vi "main.vi"() -> ()   [LabVIEW 2021]
uses:
  <vilib>/xnet/xnet.llb/XNET Frame CAN.ctl
  <vilib>/xnet/xnet.llb/XNET Frame Type CAN.ctl
  General Purpose/references.ctl
  General Purpose/measurements.ctl
  <vilib>/Platform/TimedLoop/XDataNode/timing_clust.ctl
  <vilib>/Platform/TimedLoop/XDataNode/nitl_modes.ctl
  <vilib>/Platform/TimedLoop/XDataNode/wakeup.ctl
  <instrlib>/niSync/niSync.llb/niSync Initialize (Default).vi
  <vilib>/xnet/xnet.llb/XNET Write (Frame CAN).vi
  <vilib>/xnet/xnet.llb/XNET Read (Frame CAN).vi
  <vilib>/Platform/TimedLoop/XDataNode/XDataNode.xnode
  <vilib>/Platform/TimedLoop/XDataNode/XDNodeRunTimeDep.lvlib
panel:
  out "Grandmaster Clock ID":string
  out "Synchronized":bool
  out "current time":timestamp
  in  "measurements":T1
  in  "references":T2
  out "CAN OUT":T3 {"payload" format="%x"; "timestamp" format="%<%.7X\n%x>T"; "type" items=["CAN Data"=0, "CAN Remote"=1, "CAN Bus Error"=2, "CAN 2.0 Data"=8, "CAN FD Data"=16, "CAN FD+BRS Data"=24, "J1939 Data"=192, "Delay"=224, "Log Trigger"=225, "Start Trigger"=226]; "identifier" format="%x"}
  in  "To ACT CH 4":bool
  in  "To ACT CH 3":bool
  in  "To ACT CH 2":bool
  out "Error 4":bool
  out "Fault 4":bool
  out "Error 3":bool
  out "Fault 3":bool
  out "Error 2":bool
  out "Fault 2":bool
  out "State code 4":i32
  out "State code 3":i32
  out "State code 2":i32
  out "State code 1":i32
  out "Error 1":bool
  out "Fault 1":bool
  in  "To ACT CH 1":bool
  in  "main stop":bool
  in  "Vdc4":dbl=750.0
  in  "Qac4":dbl
  in  "Vdc3":dbl=750.0
  in  "Qac3":dbl
  in  "Vdc2":dbl=750.0
  in  "Qac2":dbl
  in  "Emergency 4":bool
  in  "To IN OP  4":bool
  in  "SEND sp 4":bool
  in  "Clear 4":bool
  in  "Shutdwn 4":bool
  in  "Emergency 3":bool
  in  "To IN OP  3":bool
  in  "SEND sp 3":bool
  in  "Clear 3":bool
  in  "Shutdwn 3":bool
  in  "Emergency 2":bool
  in  "To IN OP  2":bool
  in  "SEND sp 2":bool
  in  "Clear 2":bool
  in  "Shutdwn 2":bool
  out "V slider 22":dbl(slide) caption="V-i" max=-10.0 scale=650.0..780.0 scale format="%#_4g"
  out "V slider 21":dbl(slide) caption="V-i" max=-10.0 scale=650.0..780.0 scale format="%#_4g"
  out "V slider 20":dbl(slide) caption="V-i" max=-10.0 scale=650.0..780.0 scale format="%#_4g"
  out "kW":dbl caption="Numeric" format="%#.3g"
  out "?VkVAr":dbl caption="Numeric" format="%.3g"
  out "kW":dbl caption="Numeric" format="%#.3g"
  out "?VkVAr":dbl caption="Numeric" format="%.3g"
  out "kW":dbl caption="Numeric" format="%#.3g"
  out "?VkVAr":dbl caption="Numeric" format="%.3g"
  out "OFF 4":bool
  out "ON 4":bool
  out "Ready 4":bool
  out "OFF 3":bool
  out "ON 3":bool
  out "Ready 3":bool
  out "OFF 2":bool
  out "ON 2":bool
  out "Ready 2":bool
  out "error out":errorcluster
  out "?VkVAr":dbl caption="Numeric" format="%.3g"
  out "kW":dbl caption="Numeric" format="%#.3g"
  out "V slider 19":dbl(slide) caption="V-i" max=-10.0 scale=650.0..780.0 scale format="%#_4g"
  in  "Vdc1":dbl=750.0
  out "OFF 1":bool
  out "ON 1":bool
  out "Ready 1":bool
  out "CAN IN":T3 {"payload" format="%x"; "timestamp" format="%<%.7X\n%x>T"; "type" items=["CAN Data"=0, "CAN Remote"=1, "CAN Bus Error"=2, "CAN 2.0 Data"=8, "CAN FD Data"=16, "CAN FD+BRS Data"=24, "J1939 Data"=192, "Delay"=224, "Log Trigger"=225, "Start Trigger"=226]; "identifier" format="%x"}
  in  "newfile":bool
  in  "Log period [ms]":i64=1000
  in  "Emergency 1":bool
  in  "Qac1":dbl
  in  "conv":T5
  in  "CAN [ms]":i64=1
  out "CAN with Conv":bool
  out "Measurements":bool
  in  "Shutdwn 1":bool
  in  "Clear 1":bool
  in  "SEND sp 1":bool
  in  "To IN OP 1":bool
  out "logging":bool
  # "Resource agents: AFE 1-4"
  # "package identifiers:\n1xx VSC1 \n2xx VSC2\n3xx VSC3\n4xx VSC4\n\nx0x send from agent to resource\nx02 Power setpoints\nx06 Measurements\nx9 status\n          = [state; error; alarm; OFF; Ready; ON]\n\n \n\nx1x send from resource to agent\nx10 Power measurements\nx11 Measurements\nx12 status\n          = [state; error; alarm; full; precharge; neg; 0; 0]"
  # "B18"
  # "B 22\nB19"
  # "VSC 4"
  # "B17"
  # "B21"
  # "VSC 3"
  # "B16"
  # "B20"
  # "VSC 2"
  # "B15"
  # "B19"
  # "VSC 1"
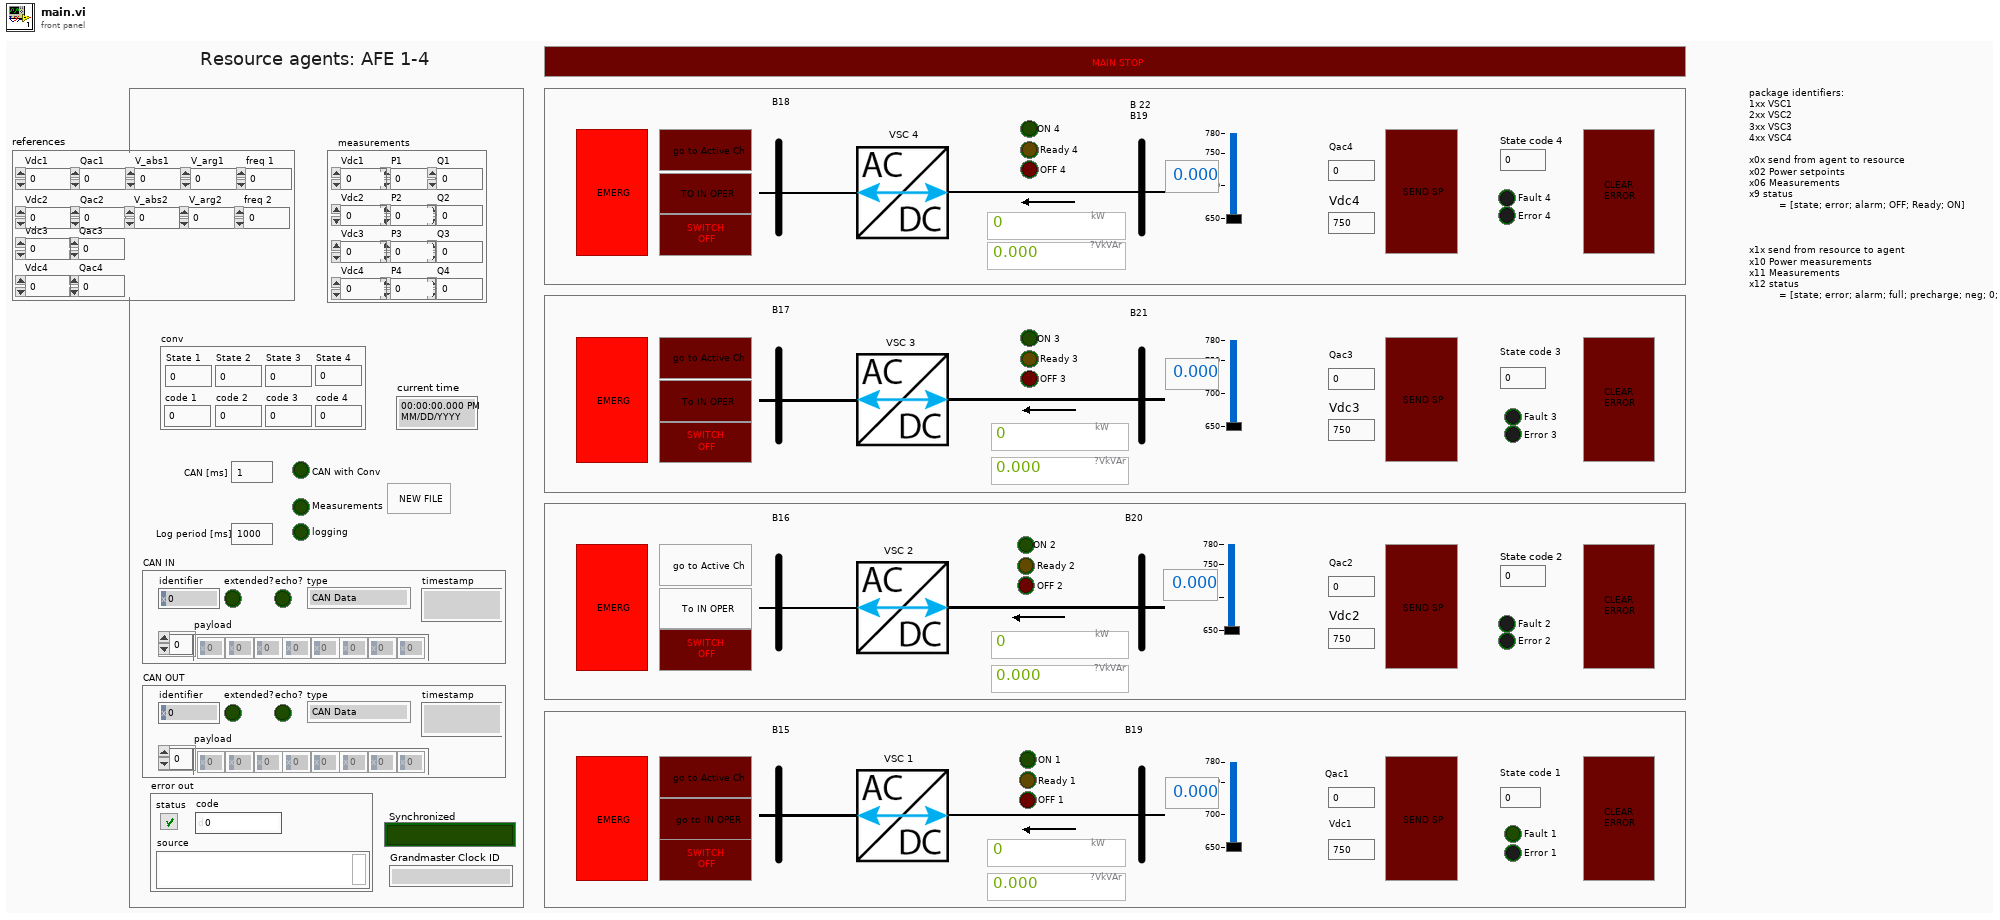
[diagram p1: front panel]
types:
  T1 = typedef "measurements.ctl" = cluster{"Vdc1":dbl, "P1":dbl, "Vdc2":dbl, "P2":dbl, "Q2":dbl, "Vdc3":dbl, "P3":dbl, "Q3":dbl, "Vdc4":dbl, "P4":dbl, "Q4":dbl, "Q1":dbl}
  T2 = typedef "references.ctl" = cluster{"Vdc1":dbl, "Vdc2":dbl, "Qac2":dbl, "Vdc3":dbl, "Qac3":dbl, "Vdc4":dbl, "Qac4":dbl, "Qac1":dbl, "V_arg2":dbl, "V_abs2":dbl, "V_abs1":dbl, "V_arg1":dbl, "freq 1":dbl, "freq 2":dbl}
  T3 = typedef "XNET Frame CAN.ctl" = cluster{"timestamp":timestamp, "payload":u8[], "identifier":u32, "type":T4, "extended?":bool, "echo?":bool}
  T4 = typedef "XNET Frame Type CAN.ctl" = u8
  T5 = cluster{"State 1":dbl, "code 1":dbl, "code 2":dbl, "code 3":dbl, "code 4":dbl, "State 2":dbl, "State 3":dbl, "State 4":dbl}
  T6 = cluster{"Frame In":refnum<k21>, "Frame Out":refnum<k21>}
  T7 = typedef "XDNodeRunTimeDep.lvlib/timing_clust.ctl" = cluster{"Expected End [f-1]":u64, "Actual End [f-1]":u64, "Finished Late? [f-1]":bool, "Expected End [i-1]":u64, "Actual End [i-1]":u64, "Finished Late? [i-1]":bool, "Expected Start [i]":u64, "Actual Start [i]":u64, "Expected Start [f]":u64, "Actual Start [f]":u64, "Source Name":string, "Structure Name":string, "Period":i64, "Deadline":i64, "Offset":i64, "Start":i64, "Priority":i32, "Timeout":i32, "Mode":T8, "Wakeup Reason":T9, "Error":errorcluster, "Source Type":string, "Secondary Source Type":string, "Global End Time":u64, "Global Start Time":u64, "Frame Duration":u64, "Iteration Duration":u64, "Assigned CPU":i32, "I/O Scan Engine Mode":u32}
  T8 = typedef "XDNodeRunTimeDep.lvlib/nitl_modes.ctl" = enum32{"No Change", "Process missed periods, maintain original phase", "Discard missed periods, maintain original phase", "Process missed periods, ignore original phase", "Discard missed periods, ignore original phase"}
  T9 = typedef "XDNodeRunTimeDep.lvlib/wakeup.ctl" = enum32{"Normal", "Aborted", "Asynchronous wakeup", "Timing source error", "Timed loop error", "Timeout"}
  T10 = cluster{"date string":string, "time string":string, "Vdc1":dbl, "P1":dbl, "Q1":dbl, "Vdc2":dbl, "P2":dbl, "Q2":dbl, "Vdc3":dbl, "P3":dbl, "Q3":dbl, "Vdc4":dbl, "P4":dbl, "Q4":dbl}
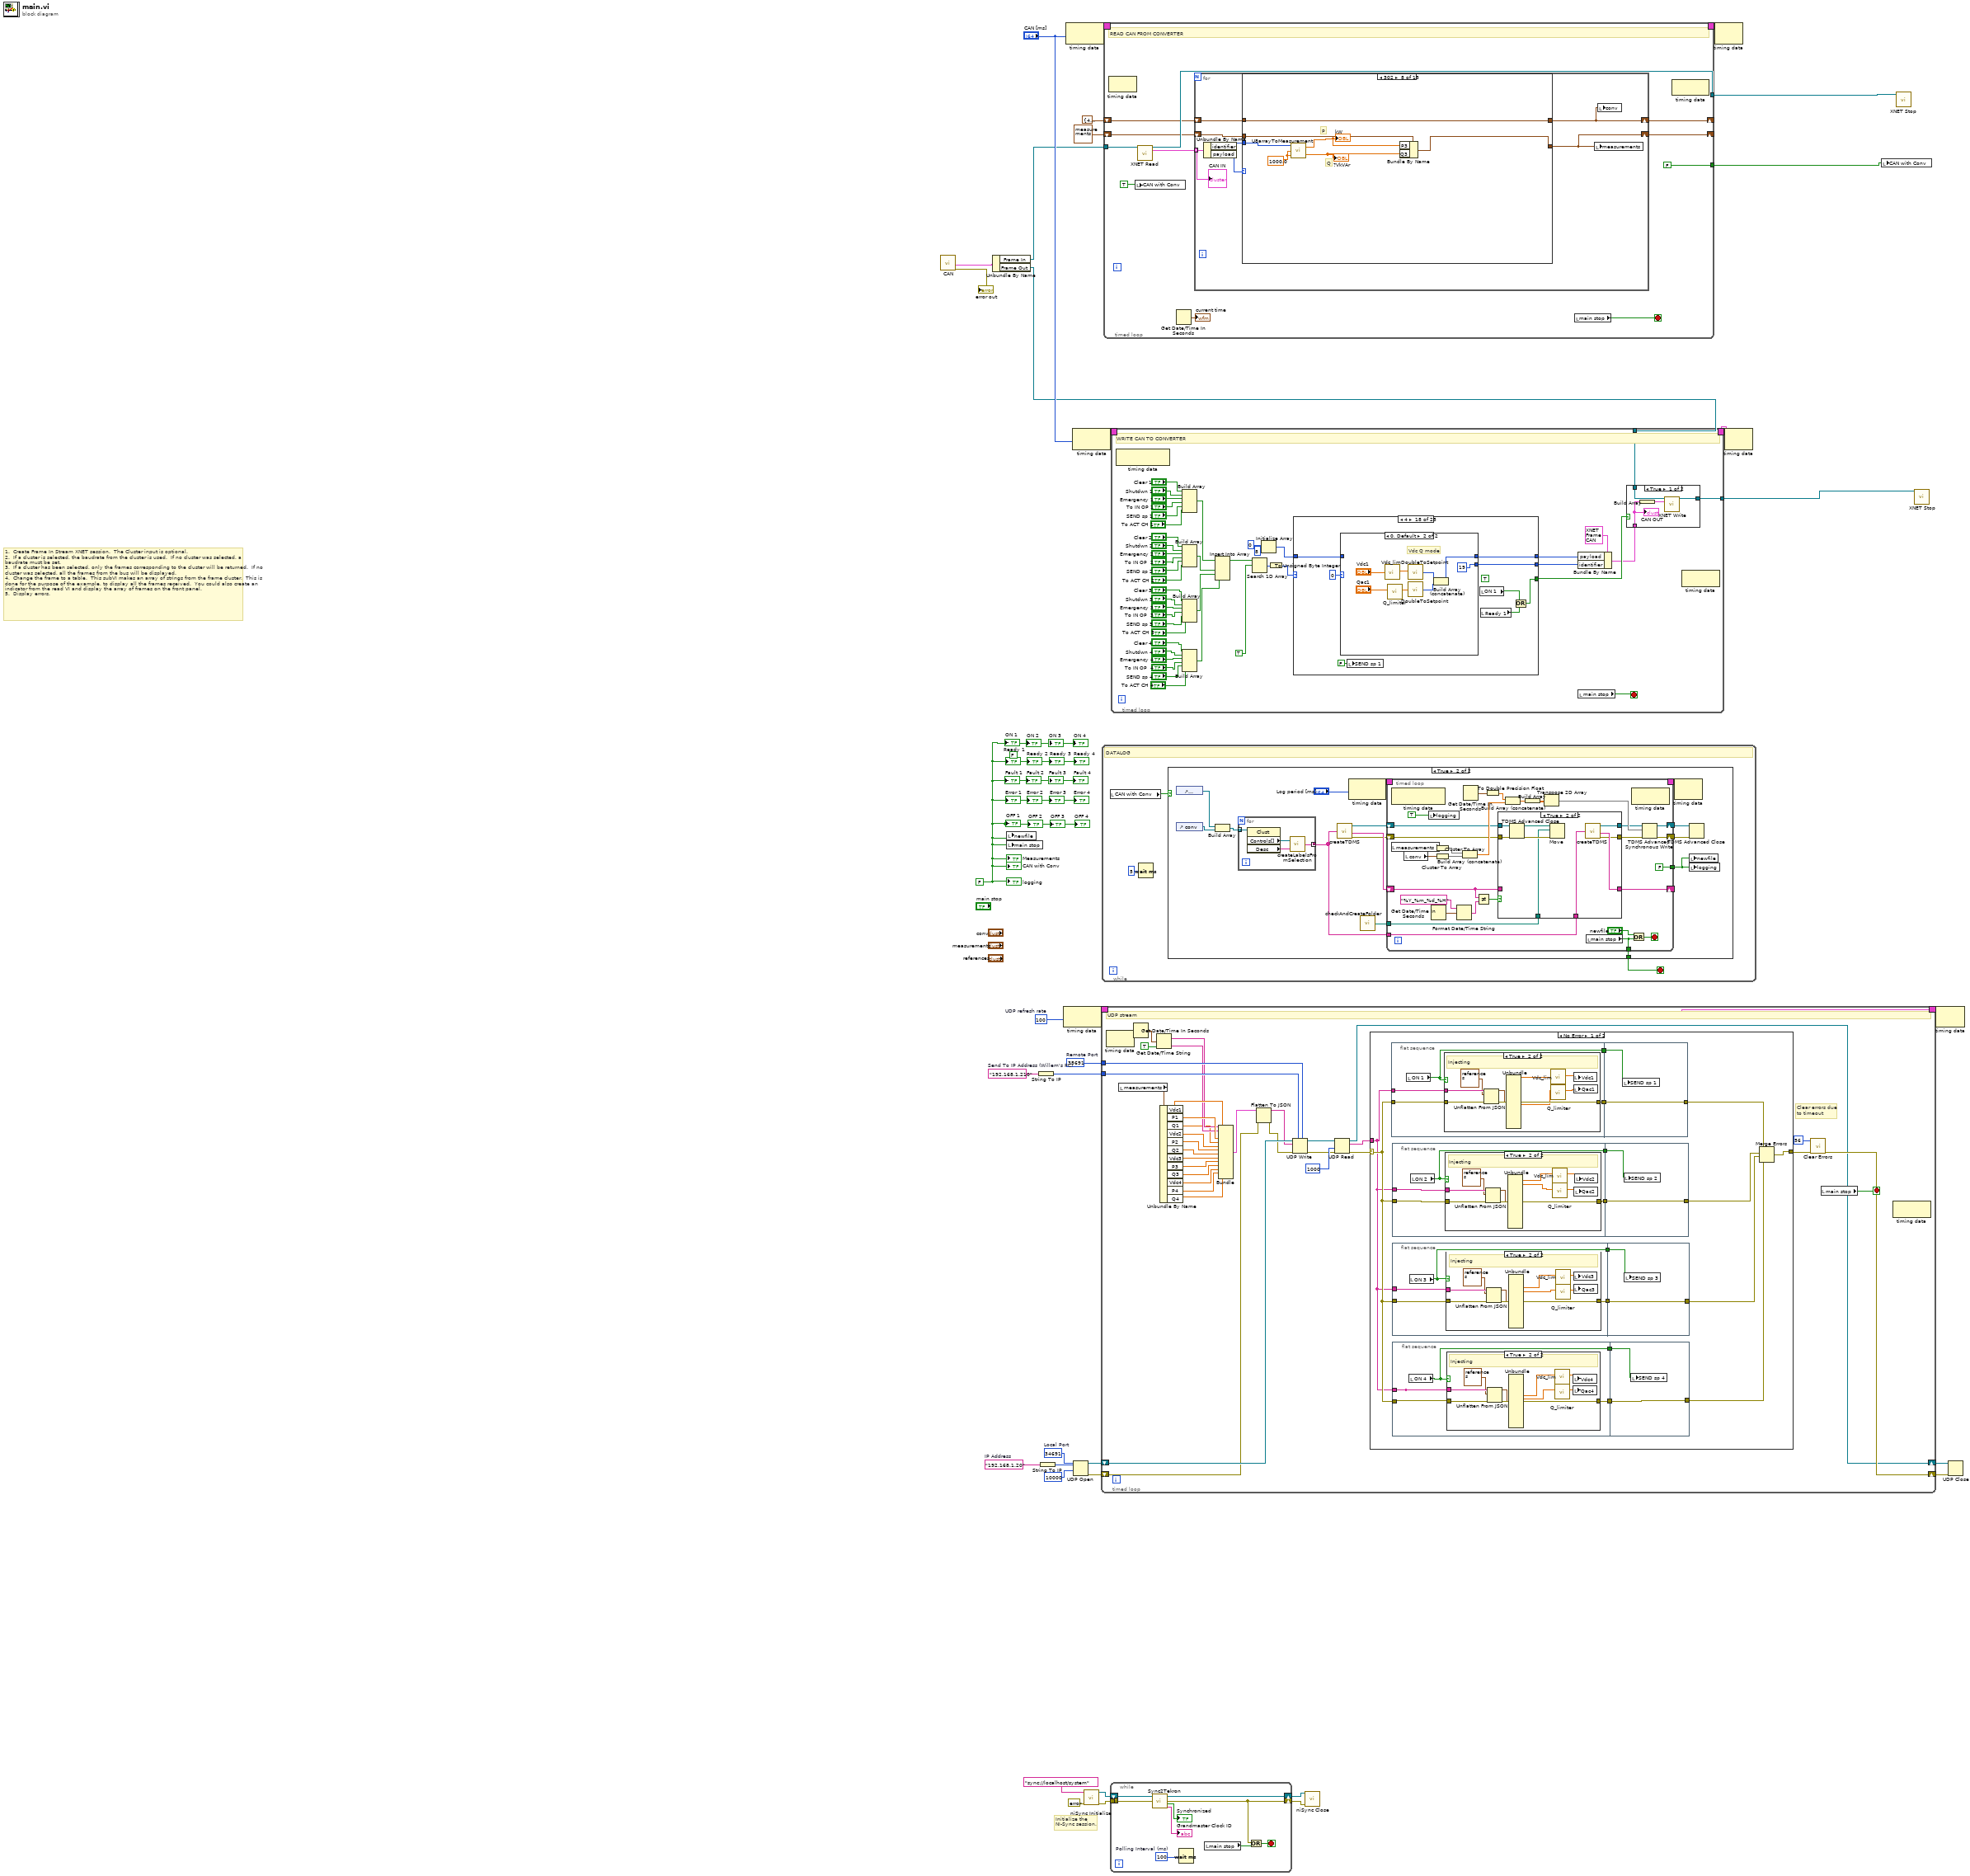
[diagram p0: block diagram]
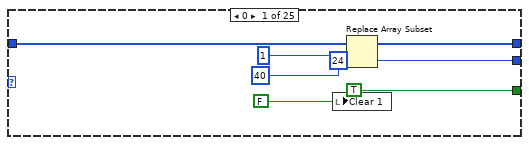
[diagram p8: hidden frame]
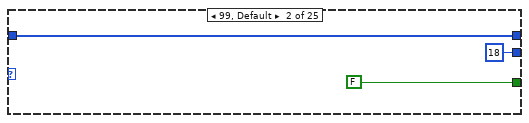
[diagram p9: hidden frame]
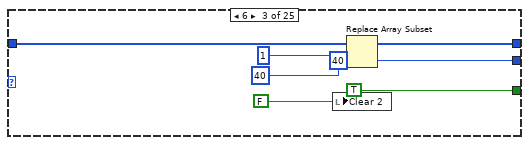
[diagram p10: hidden frame]
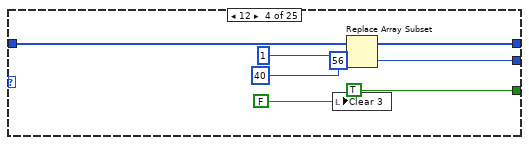
[diagram p11: hidden frame]
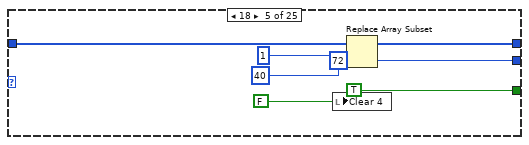
[diagram p12: hidden frame]
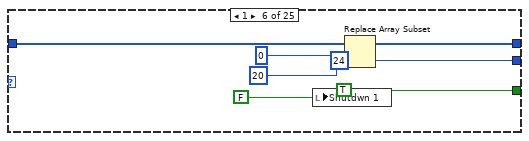
[diagram p13: hidden frame]
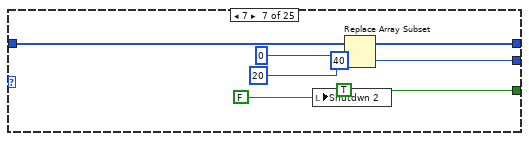
[diagram p14: hidden frame]
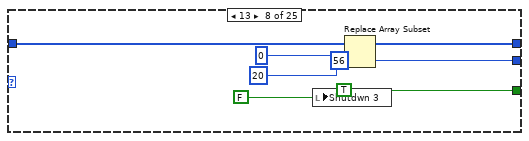
[diagram p15: hidden frame]
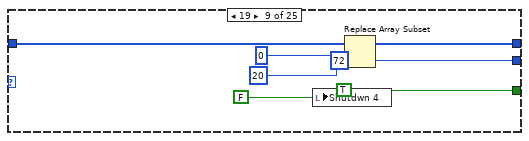
[diagram p16: hidden frame]
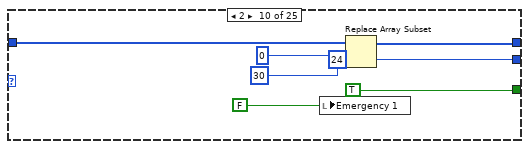
[diagram p17: hidden frame]
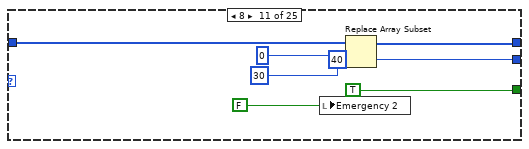
[diagram p18: hidden frame]
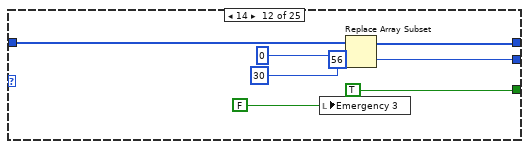
[diagram p19: hidden frame]
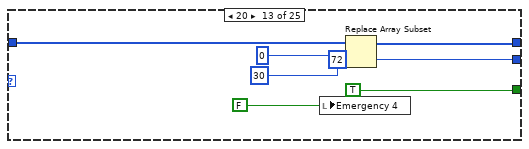
[diagram p20: hidden frame]
diagram:
  (unwired) FALSE ("ON 2")
  (unwired) FALSE ("ON 2")
  w14 = i64 100  # UDP refresh rate
  w19 = u16 34691  # Local Port
  w20 = "192.168.1.20"  # IP Address
  w10 = u16 35691  # Remote Port
  w18 = "192.168.1.210"  # Send To IP Address (Willem's PC)
  w7 = FALSE
  # "Initialize the\nNI-Sync session."
  # "1.  Create Frame In Stream XNET session.  The Cluster input is optional.  \n2.  If a cluster is selected, the baudrate from the cluster is used.  If no cluster was selected, a baudrate must be set.\n3.  If a cluster has been selected, only the frames corresponding to the cluster will be returned.  If no cluster was selected, all the frames from the bus will be displayed.\n4.  Change the frame to a table.  This subVI makes an array of strings from the frame cluster.  This is done for the purpose of the example, to display all the frames received.  You could also create an indicator from the read VI and display the array of frames on the front panel. \n5.  Display errors."
  n1 = call "CAN.vi"() -> ("error out"=→"error out":errorcluster, "CAN"=w9:T6)  [unwired: 10 in]
  n2 = Unbundle By Name(w9) -> ("Frame In"=w28:refnum<k21>, "Frame Out"=w31:refnum<k21>)
  n3 = local write "newfile"(w7) -> ()
  n4 = local write "main stop"(w7) -> ()
  n5 = String To IP(1:w18) -> (0:w11:u32)
  n6 = String To IP(1:w20) -> (0:w21:u32)
  n7 = node-c288(w14) -> (w23:T7)
  n8 = node-c288("CAN [ms]") -> (w30:T7)
  n9 = node-c288("CAN [ms]") -> (w25:T7)
  n10 = UDP Open(7:w21, 9:10000 ("timeout ms (25000)"), 11:w19) -> (port=w13:refnum<k16>, 0:w12:errorcluster)  [unwired: 2 in, 1 out]
  n11 = call-poly <instrlib>:"niSync Initialize.vi"("error in (no error)"=errorcluster {"status"=FALSE, "code"=0, "source"=""}, "resource name"=tag "sync://localhost/system" ("NI-Sync Resource")) -> ("error out"=w4:errorcluster, "instrument handle out"=w1:refnum<k15>)  [unwired: 8 in]
  n12 = timed-loop {
    timing: w23 -> [_]
    timing-out: [_] -> w22
    shift-right: [w53] -> w17
    shift-left: w13 -> [w69]
    shift-right: [w59] -> w16
    shift-left: w12 -> [w66]
    tunnel: w11 -> [w63]
    tunnel: w10 -> [w62]
    stop <- w61 stop-if-true
    # "Clear errors due\nto timeout"
    # "UDP stream"
    n13 = node-c288() -> ()  [unwired: 1 in, 1 out]
    n14 = local read "measurements"() -> (w48:T1)
    n15 = Get Date/Time In Seconds() -> (seconds since 1Jan1904=w52:timestamp)
    n16 = Get Date/Time String(seconds (now)=w52, want seconds? (F)=TRUE) -> (date string=w51:string, time string=w50:string)  [unwired: 1 in]
    n17 = Unbundle By Name(w48) -> ("Vdc1"=w68:dbl, "P1"=w67:dbl, "Q1"=w47:dbl, "Vdc2"=w46:dbl, "P2"=w44:dbl, "Q2"=w43:dbl, "Vdc3"=w42:dbl, "P3"=w41:dbl, "Q3"=w40:dbl, "Vdc4"=w39:dbl, "P4"=w38:dbl, "Q4"=w37:dbl)
    n18 = Bundle("date string"=w51, "time string"=w50, "Vdc1"=w68, "P1"=w67, "Q1"=w47, "Vdc2"=w46, "P2"=w44, "Q2"=w43, "Vdc3"=w42, "P3"=w41, "Q3"=w40, "Vdc4"=w39, "P4"=w38, "Q4"=w37) -> (w45:T10)  [unwired: 1 in]
    n19 = Flatten To JSON(anything=w45, error in (no error)=w66) -> (JSON string=w64:string, 11:w65:errorcluster)  [unwired: 1 in]
    n20 = UDP Write(address=w63, port or service name=w62, connection ID=w69, data in=w64, 8:w65) -> (error out=w55:errorcluster, 3:w54:refnum<k16>)  [unwired: 1 in]
    n21 = UDP Read(connection ID=w54, timeout ms (25000)=1000, 8:w55) -> (data out=w58:string, error out=w57:errorcluster, 3:w53:refnum<k16>)  [unwired: 1 in, 2 out]
    n22 = case shown="No Error" w57 {
      selector: w57 -> [w82 w149]
      tunnel: w58 -> [w81 _]
      tunnel: [w83 w149] -> w36
      frame No Error {
        n23 = flat-sequence {
          tunnel: w81 -> [w136]
          tunnel: w82 -> [w135]
          tunnel: [w134] -> w84
          tunnel: [w133] -> w70
          tunnel: w84 -> [w148]
          tunnel: [w148] -> w80
          tunnel: w70 -> [w147]
          frame #0 {
            n24 = local read "ON 1"() -> (w133:bool)
            n25 = case shown="True" w133 {
              tunnel: w136 -> [_ w146]
              tunnel: w135 -> [w137 w145]
              tunnel: [w137 w144] -> w134
              frame False {
                # "Injecting"
              }
              frame True {
                # "Injecting"
                n26 = Unflatten From JSON(JSON string=w146, type and defaults=T2 {"Vdc1"=0.0, "Vdc2"=0.0, "Qac2"=0.0, "Vdc3"=0.0, "Qac3"=0.0, "Vdc4"=0.0, "Qac4"=0.0, "Qac1"=0.0, "V_arg2"=0.0, "V_abs2"=0.0, "V_abs1"=0.0, "V_arg1"=0.0, "freq 1"=0.0, "freq 2"=0.0} ("ref"), error in (no error)=w145) -> (value=w143:T2, error out=w144:errorcluster)  [unwired: 4 in]
                n27 = Unbundle(w143) -> ("Vdc1"=w140:dbl, "Qac1"=w138:dbl)  [unwired: 12 out]
                n28 = call "Vdc_lim.vi"("IN Vdc"=w140) -> ("OUT Vdc"=w141:dbl)  [unwired: 10 in]
                n29 = call "Q_limiter.vi"("IN Q"=w138) -> ("OUT Q"=w139:dbl)  [unwired: 10 in]
                n30 = local write "Vdc1"(w141) -> ()
                n31 = local write "Qac1"(w139) -> ()
              }
            }
          }
          frame #1 {
            n32 = local write "SEND sp 1"(w147) -> ()
          }
        }
        n33 = flat-sequence {
          tunnel: w82 -> [w120]
          tunnel: w81 -> [w118]
          tunnel: [w119] -> w74
          tunnel: [w117] -> w71
          tunnel: [w132] -> w77
          tunnel: w74 -> [w132]
          tunnel: w71 -> [w131]
          frame #0 {
            n34 = local read "ON 2"() -> (w117:bool)
            n35 = case shown="True" w117 {
              tunnel: w118 -> [_ w130]
              tunnel: w120 -> [w121 w129]
              tunnel: [w121 w128] -> w119
              frame False {
                # "Injecting"
              }
              frame True {
                # "Injecting"
                n36 = Unflatten From JSON(JSON string=w130, type and defaults=T2 {"Vdc1"=0.0, "Vdc2"=0.0, "Qac2"=0.0, "Vdc3"=0.0, "Qac3"=0.0, "Vdc4"=0.0, "Qac4"=0.0, "Qac1"=0.0, "V_arg2"=0.0, "V_abs2"=0.0, "V_abs1"=0.0, "V_arg1"=0.0, "freq 1"=0.0, "freq 2"=0.0} ("ref"), error in (no error)=w129) -> (value=w127:T2, error out=w128:errorcluster)  [unwired: 4 in]
                n37 = Unbundle(w127) -> ("Vdc2"=w124:dbl, "Qac2"=w122:dbl)  [unwired: 12 out]
                n38 = call "Vdc_lim.vi"("IN Vdc"=w124) -> ("OUT Vdc"=w125:dbl)  [unwired: 10 in]
                n39 = call "Q_limiter.vi"("IN Q"=w122) -> ("OUT Q"=w123:dbl)  [unwired: 10 in]
                n40 = local write "Qac2"(w123) -> ()
                n41 = local write "Vdc2"(w125) -> ()
              }
            }
          }
          frame #1 {
            n42 = local write "SEND sp 2"(w131) -> ()
          }
        }
        n43 = flat-sequence {
          tunnel: w82 -> [w104]
          tunnel: w81 -> [w102]
          tunnel: [w103] -> w75
          tunnel: [w101] -> w72
          tunnel: [w116] -> w78
          tunnel: w75 -> [w116]
          tunnel: w72 -> [w115]
          frame #0 {
            n44 = local read "ON 3"() -> (w101:bool)
            n45 = case shown="True" w101 {
              tunnel: w102 -> [_ w114]
              tunnel: w104 -> [w105 w113]
              tunnel: [w105 w112] -> w103
              frame False {
                # "Injecting"
              }
              frame True {
                # "Injecting"
                n46 = Unflatten From JSON(JSON string=w114, type and defaults=T2 {"Vdc1"=0.0, "Vdc2"=0.0, "Qac2"=0.0, "Vdc3"=0.0, "Qac3"=0.0, "Vdc4"=0.0, "Qac4"=0.0, "Qac1"=0.0, "V_arg2"=0.0, "V_abs2"=0.0, "V_abs1"=0.0, "V_arg1"=0.0, "freq 1"=0.0, "freq 2"=0.0} ("ref"), error in (no error)=w113) -> (value=w111:T2, error out=w112:errorcluster)  [unwired: 4 in]
                n47 = Unbundle(w111) -> ("Vdc3"=w108:dbl, "Qac3"=w106:dbl)  [unwired: 12 out]
                n48 = call "Vdc_lim.vi"("IN Vdc"=w108) -> ("OUT Vdc"=w109:dbl)  [unwired: 10 in]
                n49 = call "Q_limiter.vi"("IN Q"=w106) -> ("OUT Q"=w107:dbl)  [unwired: 10 in]
                n50 = local write "Vdc3"(w109) -> ()
                n51 = local write "Qac3"(w107) -> ()
              }
            }
          }
          frame #1 {
            n52 = local write "SEND sp 3"(w115) -> ()
          }
        }
        n53 = flat-sequence {
          tunnel: w82 -> [w88]
          tunnel: [w86] -> _
          tunnel: w81 -> [w86]
          tunnel: [w87] -> w76
          tunnel: [w85] -> w73
          tunnel: [w100] -> w79
          tunnel: w76 -> [w100]
          tunnel: w73 -> [w99]
          frame #0 {
            n54 = local read "ON 4"() -> (w85:bool)
            n55 = case shown="True" w85 {
              tunnel: w86 -> [_ w98]
              tunnel: w88 -> [w89 w97]
              tunnel: [w89 w96] -> w87
              frame False {
                # "Injecting"
              }
              frame True {
                # "Injecting"
                n56 = Unflatten From JSON(JSON string=w98, type and defaults=T2 {"Vdc1"=0.0, "Vdc2"=0.0, "Qac2"=0.0, "Vdc3"=0.0, "Qac3"=0.0, "Vdc4"=0.0, "Qac4"=0.0, "Qac1"=0.0, "V_arg2"=0.0, "V_abs2"=0.0, "V_abs1"=0.0, "V_arg1"=0.0, "freq 1"=0.0, "freq 2"=0.0} ("ref"), error in (no error)=w97) -> (value=w95:T2, error out=w96:errorcluster)  [unwired: 4 in]
                n57 = Unbundle(w95) -> ("Vdc4"=w92:dbl, "Qac4"=w91:dbl)  [unwired: 12 out]
                n58 = call "Vdc_lim.vi"("IN Vdc"=w92) -> ("OUT Vdc"=w93:dbl)  [unwired: 10 in]
                n59 = call "Q_limiter.vi"("IN Q"=w91) -> ("OUT Q"=w90:dbl)  [unwired: 10 in]
                n60 = local write "Vdc4"(w93) -> ()
                n61 = local write "Qac4"(w90) -> ()
              }
            }
          }
          frame #1 {
            n62 = local write "SEND sp 4"(w99) -> ()
          }
        }
        n63 = Merge Errors(w80, w77, w78, w79) -> (w83:errorcluster)
      }
      frame Error {
      }
    }
    n64 = call <vilib>:"Clear Errors.vi"("error in (no error)"=w36, "specific error code to clear (0: all)"=56) -> ("error out"=w59:errorcluster)  [unwired: 4 in, 1 out]
    n65 = local read "main stop"() -> (w61:bool)
    n66 = node-c288() -> ()  [unwired: 1 in, 1 out]
  }
  n67 = while {
    stop <- w154 stop-if-true
    # "DATALOG"
    n68 = local read "CAN with Conv"() -> (w152:bool)
    n69 = Wait (ms)(milliseconds to wait=u32 5) -> ()  [unwired: 1 out]
    n70 = case shown="True" w152 {
      selector: w152 -> [w155 _]
      tunnel: [w155 w168] -> w154
      frame False {
      }
      frame True {
        n71 = control-ref of="measurements"() -> (w156:refnum<vi>)
        n72 = control-ref of="conv"() -> (w161:refnum<vi>)
        n73 = Build Array(w156, w161) -> (w160:refnum<vi>[])
        n74 = for {
          tunnel: [w172] -> w159 mode=concatenating
          tunnel: w160 -> [w171] mode=indexing
          n75 = property class="Clust"(reference=w171) -> ("Controls[]"=w174:refnum<vi>[], "Desc"=w173:string)  [unwired: 1 in, 2 out]
          n76 = call "createLabelsFromSelection.vi"("log_from"=w173, "Controls[]"=w174) -> ("labels_to_log"=w172:string[])
        }
        n77 = call "createTDMS.vi"("channel name(s)"=w159) -> ("Ref"=w157:refnum<k34>, "hour"=w163:string, "error out"=w158:errorcluster)  [unwired: 3 in]
        n78 = node-c288("Log period [ms]") -> (w170:T7)
        n79 = call "checkAndCreateFolder.vi"() -> ("dup path"=w162:path)  [unwired: 1 in]
        n80 = timed-loop {
          timing: w170 -> [_]
          timing-out: [_] -> w169
          tunnel: [w194] -> w168
          tunnel: [FALSE ("logging")] -> w164
          shift-right: [w185] -> _
          shift-left: w163 -> [w184]
          tunnel: w162 -> [w183]
          tunnel: w159 -> [w182]
          shift-right: [w195] -> w165
          shift-left: w158 -> [w176]
          shift-right: [w203] -> w166
          shift-left: w157 -> [w175]
          stop <- w197 stop-if-true
          n81 = node-c288() -> ()  [unwired: 1 in, 1 out]
          n82 = local read "measurements"() -> (w181:T1)
          n83 = local read "conv"() -> (w180:T5)
          n84 = local write "logging"(TRUE ("logging")) -> ()
          n85 = Get Date/Time In Seconds() -> (seconds since 1Jan1904=w188:timestamp)
          n86 = Cluster To Array(cluster=w181) -> (array=w179:dbl[])
          n87 = Cluster To Array(cluster=w180) -> (array=w178:dbl[])
          n88 = Format Date/Time String(time format string (%c)="%Y_%m_%d_%H", seconds (now)=w188) -> (date/time string=w186:string)  [unwired: 1 in]
          n89 = Build Array (concatenate)(w179, w178) -> (w177:dbl[])
          n90 = Get Date/Time In Seconds() -> (seconds since 1Jan1904=w199:timestamp)
          n91 = Not Equal?(x=w184, y=w186) -> (x != y?=w187:bool)
          n92 = To Double Precision Float(number=w199) -> (double precision float=w198:dbl)
          n93 = case shown="True" w187 {
            tunnel: w175 -> [w206 w215]
            tunnel: [w206 w209] -> w191
            tunnel: w176 -> [w205 w214]
            tunnel: [w205 w207] -> w190
            tunnel: [w204 w208] -> w185
            tunnel: w184 -> [w204 _]
            tunnel: w183 -> [_ w211]
            tunnel: w182 -> [_ w210]
            frame False {
            }
            frame True {
              n94 = TDMS Advanced Close(8:w214, 11:w215) -> (0:w213:errorcluster, 3:w212:path)  [unwired: 2 in]
              n95 = Move(source path=w212, error in=w213, 10:w211) -> ()  [unwired: 2 in, 3 out]
              n96 = call "createTDMS.vi"("channel name(s)"=w210) -> ("Ref"=w209:refnum<k34>, "hour"=w208:string, "error out"=w207:errorcluster)  [unwired: 3 in]
            }
          }
          n97 = Build Array (concatenate)(w198, w177) -> (w202:dbl[])
          n98 = Build Array(w202) -> (w201:dbl[][])
          n99 = Transpose 2D Array(2D array=w201) -> (transposed array=w200:dbl[][])
          n100 = local read "main stop"() -> (w194:bool)
          n101 = node-c288() -> ()  [unwired: 1 in, 1 out]
          n102 = Or(x="newfile", y=w194) -> (x .or. y?=w197:bool)
          n103 = TDMS Advanced Synchronous Write(8:w190, 10:w200, 11:w191) -> (0:w195:errorcluster, 3:w203:refnum<k34>)
        }
        n104 = node-c288(w169) -> ()  [unwired: 1 out]
        n105 = TDMS Advanced Close(8:w165, 11:w166) -> ()  [unwired: 2 in, 2 out]
        n106 = local write "newfile"(w164) -> ()
        n107 = local write "logging"(w164) -> ()
      }
    }
  }
  n108 = timed-loop {
    timing: w30 -> [_]
    timing-out: [_] -> w29
    tunnel: w28 -> [w225]
    tunnel: [w231] -> w35
    shift-right: [w226] -> _
    shift-left: T5 {"State 1"=4.0, "code 1"=0.0, "code 2"=0.0, "code 3"=0.0, "code 4"=0.0, "State 2"=4.0, "State 3"=4.0, "State 4"=4.0} ("Conv 2") -> [w230]
    tunnel: [FALSE ("stop CAN")] -> w32
    shift-right: [w223] -> _
    shift-left: T1 {"Vdc1"=0.0, "P1"=0.0, "Vdc2"=0.0, "P2"=0.0, "Q2"=0.0, "Vdc3"=0.0, "P3"=0.0, "Q3"=0.0, "Vdc4"=0.0, "P4"=0.0, "Q4"=0.0, "Q1"=0.0} ("measurements 2") -> [w224]
    stop <- w229 stop-if-true
    # "READ CAN FROM CONVERTER"
    n109 = node-c288() -> ()  [unwired: 1 in, 1 out]
    n110 = local write "CAN with Conv"(TRUE) -> ()
    n111 = call-poly <vilib>:"XNET Read.vi"("session in"=w225) -> ("session out"=w231:refnum<k21>, "data"=w232:T3[])  [unwired: 11 in, 2 out]
    n112 = Get Date/Time In Seconds() -> (seconds since 1Jan1904=→"current time":timestamp)
    n113 = for {
      tunnel: w232 -> [w237] mode=indexing
      shift-right: [w235] -> w226
      shift-left: w230 -> [w236]
      shift-right: [w233] -> w223
      shift-left: w224 -> [w234]
      n114 = Unbundle By Name(w237) -> ("identifier"=w239:u32, "payload"=w238:u8[])
      n115 = case shown="302" w239 {
        tunnel: w238 -> [_ w246 w271 w296 w321 w348 w355 w362 w369 w374 w382 w390 w398]
        tunnel: w236 -> [w241 w254 w279 w304 w329 w346 w353 w360 w367 w372 w378 w387 w395]
        tunnel: [w241 w253 w278 w303 w328 w346 w353 w360 w367 w372 w378 w387 w395] -> w235
        tunnel: w234 -> [w240 w243 w268 w293 w319 w344 w349 w356 w363 w370 w377 w386 w393]
        tunnel: [w240 w244 w269 w294 w320 w345 w350 w357 w364 w371 w376 w385 w394] -> w233
        frame 0, Default {
        }
        frame 25 {
          w242 = 1.0 ("factor 1")
          n116 = Index Array(array=w246, index=0) -> (element=w247:u8)
          n117 = call "U8arrayToMeasurement.vi"("factor 2"=w242, "factor 1"=w242, "payload"=w246) -> ("Meas 2"=w245:dbl)  [unwired: 1 out]
          "V slider 19" <- w245
          n118 = Index Array(array=w246, index=1) -> (element=w250:u8)
          n119 = Index Array(array=w246, index=2) -> (element=w249:u8)
          n120 = Join Numbers(hi=w250, lo=w249) -> ((hi.lo)=w248:u16)
          "State code 1" <- w248
          n121 = Bundle By Name(cluster=w243, "Vdc1"=w245) -> (w244:T1)
          n122 = case shown="5" w247 {
            frame 5 {
              w257 = FALSE ("Fault 1")
              n123 = local write "Fault 1"(TRUE ("Fault 1")) -> ()
              n124 = local write "Error 1"(w257) -> ()
              n125 = local write "OFF 1"(w257) -> ()
              n126 = local write "Ready 1"(w257) -> ()
              n127 = local write "ON 1"(w257) -> ()
            }
            frame 1 {
              w258 = FALSE ("Fault 1")
              n128 = local write "Fault 1"(w258) -> ()
              n129 = local write "Error 1"(TRUE ("Error 1")) -> ()
              n130 = local write "OFF 1"(w258) -> ()
              n131 = local write "Ready 1"(w258) -> ()
              n132 = local write "ON 1"(w258) -> ()
            }
            frame 2 {
              w261 = FALSE ("Fault 1")
              n133 = local write "Fault 1"(w261) -> ()
              n134 = local write "Error 1"(w261) -> ()
              n135 = local write "OFF 1"(TRUE ("OFF 1")) -> ()
              n136 = local write "Ready 1"(w261) -> ()
              n137 = local write "ON 1"(w261) -> ()
            }
            frame 3 {
              w263 = FALSE ("Fault 1")
              n138 = local write "Fault 1"(w263) -> ()
              n139 = local write "Error 1"(w263) -> ()
              n140 = local write "OFF 1"(w263) -> ()
              n141 = local write "Ready 1"(TRUE ("Ready 1")) -> ()
              n142 = local write "ON 1"(w263) -> ()
            }
            frame 4 {
              w265 = FALSE ("Fault 1")
              n143 = local write "Fault 1"(w265) -> ()
              n144 = local write "Error 1"(w265) -> ()
              n145 = local write "OFF 1"(w265) -> ()
              n146 = local write "Ready 1"(w265) -> ()
              n147 = local write "ON 1"(TRUE ("ON 1")) -> ()
            }
            frame 99, Default {
              w266 = FALSE ("Fault 1")
              n148 = local write "Fault 1"(w266) -> ()
              n149 = local write "Error 1"(w266) -> ()
              n150 = local write "OFF 1"(w266) -> ()
              n151 = local write "Ready 1"(w266) -> ()
              n152 = local write "ON 1"(w266) -> ()
            }
          }
          n153 = Bundle By Name(cluster=w254, "State 1"=w247, "code 1"=w248) -> (w253:T5)
        }
        frame 41 {
          w267 = 1.0 ("factor 1")
          n154 = call "U8arrayToMeasurement.vi"("factor 2"=w267, "factor 1"=w267, "payload"=w271) -> ("Meas 2"=w270:dbl)  [unwired: 1 out]
          "V slider 20" <- w270
          n155 = Index Array(array=w271, index=0) -> (element=w277:u8)
          n156 = Index Array(array=w271, index=1) -> (element=w274:u8)
          n157 = Index Array(array=w271, index=2) -> (element=w273:u8)
          n158 = Join Numbers(hi=w274, lo=w273) -> ((hi.lo)=w272:u16)
          "State code 2" <- w272
          n159 = Bundle By Name(cluster=w268, "Vdc2"=w270) -> (w269:T1)
          n160 = case shown="5" w277 {
            frame 5 {
              w282 = FALSE ("Fault 1")
              n161 = local write "Fault 2"(TRUE ("Fault 1")) -> ()
              n162 = local write "Error 2"(w282) -> ()
              n163 = local write "OFF 2"(w282) -> ()
              n164 = local write "Ready 2"(w282) -> ()
              n165 = local write "ON 2"(w282) -> ()
            }
            frame 1 {
              w283 = FALSE ("Fault 1")
              n166 = local write "Fault 2"(w283) -> ()
              n167 = local write "Error 2"(TRUE ("Error 1")) -> ()
              n168 = local write "OFF 2"(w283) -> ()
              n169 = local write "Ready 2"(w283) -> ()
              n170 = local write "ON 2"(w283) -> ()
            }
            frame 2 {
              w286 = FALSE ("Fault 1")
              n171 = local write "Fault 2"(w286) -> ()
              n172 = local write "Error 2"(w286) -> ()
              n173 = local write "OFF 2"(TRUE ("OFF 1")) -> ()
              n174 = local write "Ready 2"(w286) -> ()
              n175 = local write "ON 2"(w286) -> ()
            }
            frame 3 {
              w288 = FALSE ("Fault 1")
              n176 = local write "Fault 2"(w288) -> ()
              n177 = local write "Error 2"(w288) -> ()
              n178 = local write "OFF 2"(w288) -> ()
              n179 = local write "Ready 2"(TRUE ("Ready 1")) -> ()
              n180 = local write "ON 2"(w288) -> ()
            }
            frame 4 {
              w290 = FALSE ("Fault 1")
              n181 = local write "Fault 2"(w290) -> ()
              n182 = local write "Error 2"(w290) -> ()
              n183 = local write "OFF 2"(w290) -> ()
              n184 = local write "Ready 2"(w290) -> ()
              n185 = local write "ON 2"(TRUE ("ON 1")) -> ()
            }
            frame 99, Default {
              w291 = FALSE ("Fault 1")
              n186 = local write "Fault 2"(w291) -> ()
              n187 = local write "Error 2"(w291) -> ()
              n188 = local write "OFF 2"(w291) -> ()
              n189 = local write "Ready 2"(w291) -> ()
              n190 = local write "ON 2"(w291) -> ()
            }
          }
          n191 = Bundle By Name(cluster=w279, "State 2"=w277, "code 2"=w272) -> (w278:T5)
        }
        frame 57 {
          w292 = 1.0 ("factor 1")
          n192 = Index Array(array=w296, index=0) -> (element=w302:u8)
          n193 = Index Array(array=w296, index=1) -> (element=w299:u8)
          n194 = Index Array(array=w296, index=2) -> (element=w298:u8)
          n195 = call "U8arrayToMeasurement.vi"("factor 2"=w292, "factor 1"=w292, "payload"=w296) -> ("Meas 2"=w295:dbl)  [unwired: 1 out]
          "V slider 21" <- w295
          n196 = Join Numbers(hi=w299, lo=w298) -> ((hi.lo)=w297:u16)
          "State code 3" <- w297
          n197 = case shown="5" w302 {
            frame 5 {
              w307 = FALSE ("Fault 1")
              n198 = local write "Fault 3"(TRUE ("Fault 1")) -> ()
              n199 = local write "Error 3"(w307) -> ()
              n200 = local write "OFF 3"(w307) -> ()
              n201 = local write "Ready 3"(w307) -> ()
              n202 = local write "ON 3"(w307) -> ()
            }
            frame 1 {
              w308 = FALSE ("Fault 1")
              n203 = local write "Fault 3"(w308) -> ()
              n204 = local write "Error 3"(TRUE ("Error 1")) -> ()
              n205 = local write "OFF 3"(w308) -> ()
              n206 = local write "Ready 3"(w308) -> ()
              n207 = local write "ON 3"(w308) -> ()
            }
            frame 2 {
              w311 = FALSE ("Fault 1")
              n208 = local write "Fault 3"(w311) -> ()
              n209 = local write "Error 3"(w311) -> ()
              n210 = local write "OFF 3"(TRUE ("OFF 1")) -> ()
              n211 = local write "Ready 3"(w311) -> ()
              n212 = local write "ON 3"(w311) -> ()
            }
            frame 3 {
              w313 = FALSE ("Fault 1")
              n213 = local write "Fault 3"(w313) -> ()
              n214 = local write "Error 3"(w313) -> ()
              n215 = local write "OFF 3"(w313) -> ()
              n216 = local write "Ready 3"(TRUE ("Ready 1")) -> ()
              n217 = local write "ON 3"(w313) -> ()
            }
            frame 4 {
              w315 = FALSE ("Fault 1")
              n218 = local write "Fault 3"(w315) -> ()
              n219 = local write "Error 3"(w315) -> ()
              n220 = local write "OFF 3"(w315) -> ()
              n221 = local write "Ready 3"(w315) -> ()
              n222 = local write "ON 3"(TRUE ("ON 1")) -> ()
            }
            frame 99, Default {
              w316 = FALSE ("Fault 1")
              n223 = local write "Fault 3"(w316) -> ()
              n224 = local write "Error 3"(w316) -> ()
              n225 = local write "OFF 3"(w316) -> ()
              n226 = local write "Ready 3"(w316) -> ()
              n227 = local write "ON 3"(w316) -> ()
            }
          }
          n228 = Bundle By Name(cluster=w293, "Vdc3"=w295) -> (w294:T1)
          n229 = Bundle By Name(cluster=w304, "State 3"=w302, "code 3"=w297) -> (w303:T5)
        }
        frame 73 {
          w317 = 1.0 ("factor 1")
          n230 = Index Array(array=w321, index=0) -> (element=w327:u8)
          n231 = Index Array(array=w321, index=1) -> (element=w324:u8)
          n232 = Index Array(array=w321, index=2) -> (element=w323:u8)
          n233 = Join Numbers(hi=w324, lo=w323) -> ((hi.lo)=w322:u16)
          "State code 4" <- w322
          n234 = call "U8arrayToMeasurement.vi"("factor 2"=w317, "factor 1"=w317, "payload"=w321) -> ("Meas 2"=w318:dbl)  [unwired: 1 out]
          "V slider 22" <- w318
          n235 = case shown="5" w327 {
            frame 5 {
              w332 = FALSE ("Fault 1")
              n236 = local write "Fault 4"(TRUE ("Fault 1")) -> ()
              n237 = local write "Error 4"(w332) -> ()
              n238 = local write "OFF 4"(w332) -> ()
              n239 = local write "Ready 4"(w332) -> ()
              n240 = local write "ON 4"(w332) -> ()
            }
            frame 1 {
              w333 = FALSE ("Fault 1")
              n241 = local write "Fault 4"(w333) -> ()
              n242 = local write "Error 4"(TRUE ("Error 1")) -> ()
              n243 = local write "OFF 4"(w333) -> ()
              n244 = local write "Ready 4"(w333) -> ()
              n245 = local write "ON 4"(w333) -> ()
            }
            frame 2 {
              w336 = FALSE ("Fault 1")
              n246 = local write "Fault 4"(w336) -> ()
              n247 = local write "Error 4"(w336) -> ()
              n248 = local write "OFF 4"(TRUE ("OFF 1")) -> ()
              n249 = local write "Ready 4"(w336) -> ()
              n250 = local write "ON 4"(w336) -> ()
            }
            frame 3 {
              w338 = FALSE ("Fault 1")
              n251 = local write "Fault 4"(w338) -> ()
              n252 = local write "Error 4"(w338) -> ()
              n253 = local write "OFF 4"(w338) -> ()
              n254 = local write "Ready 4"(TRUE ("Ready 1")) -> ()
              n255 = local write "ON 4"(w338) -> ()
            }
            frame 4 {
              w340 = FALSE ("Fault 1")
              n256 = local write "Fault 4"(w340) -> ()
              n257 = local write "Error 4"(w340) -> ()
              n258 = local write "OFF 4"(w340) -> ()
              n259 = local write "Ready 4"(w340) -> ()
              n260 = local write "ON 4"(TRUE ("ON 1")) -> ()
            }
            frame 99, Default {
              w341 = FALSE ("Fault 1")
              n261 = local write "Fault 4"(w341) -> ()
              n262 = local write "Error 4"(w341) -> ()
              n263 = local write "OFF 4"(w341) -> ()
              n264 = local write "Ready 4"(w341) -> ()
              n265 = local write "ON 4"(w341) -> ()
            }
          }
          n266 = Bundle By Name(cluster=w319, "Vdc4"=w318) -> (w320:T1)
          n267 = Bundle By Name(cluster=w329, "State 4"=w327, "code 4"=w322) -> (w328:T5)
        }
        frame 258 {
          w347 = 1000.0 ("factor 1")
          # "Q"
          # "P"
          n268 = call "U8arrayToMeasurement.vi"("factor 2"=w347, "factor 1"=w347, "payload"=w348) -> ("Meas 2"=w342:dbl, "Meas 1"=w343:dbl)
          "kW" <- w343
          "?VkVAr" <- w342
          n269 = Bundle By Name(cluster=w344, "P1"=w343, "Q1"=w342) -> (w345:T1)
        }
        frame 514 {
          w354 = 1000.0 ("factor 1")
          # "Q"
          # "P"
          n270 = call "U8arrayToMeasurement.vi"("factor 2"=w354, "factor 1"=w354, "payload"=w355) -> ("Meas 2"=w351:dbl, "Meas 1"=w352:dbl)
          "kW" <- w352
          "?VkVAr" <- w351
          n271 = Bundle By Name(cluster=w349, "P2"=w352, "Q2"=w351) -> (w350:T1)
        }
        frame 770 {
          w361 = 1000.0 ("factor 1")
          # "Q"
          # "P"
          n272 = call "U8arrayToMeasurement.vi"("factor 2"=w361, "factor 1"=w361, "payload"=w362) -> ("Meas 2"=w358:dbl, "Meas 1"=w359:dbl)
          "kW" <- w359
          "?VkVAr" <- w358
          n273 = Bundle By Name(cluster=w356, "P3"=w359, "Q3"=w358) -> (w357:T1)
        }
        frame 1026 {
          w368 = 1000.0 ("factor 1")
          # "Q"
          # "P"
          n274 = call "U8arrayToMeasurement.vi"("factor 2"=w368, "factor 1"=w368, "payload"=w369) -> ("Meas 2"=w365:dbl, "Meas 1"=w366:dbl)
          "kW" <- w366
          "?VkVAr" <- w365
          n275 = Bundle By Name(cluster=w363, "P4"=w366, "Q4"=w365) -> (w364:T1)
        }
        frame 262 {
          w375 = 1.0 ("factor 1")
          n276 = call "U8arrayToMeasurement.vi"("factor 2"=w375, "factor 1"=w375, "payload"=w374) -> ("Meas 1"=w373:dbl)  [unwired: 1 out]
          n277 = Bundle By Name(cluster=w370, "Vdc1"=w373) -> (w371:T1)
        }
        frame 518 {
          w383 = 1.0 ("factor 1")
          # "Vdc"
          n278 = call "U8arrayToMeasurement.vi"("factor 2"=w383, "factor 1"=w383, "payload"=w382) -> ("Meas 2"=w380:dbl, "Meas 1"=w381:dbl)
          n279 = Add(x=w381, y=w380) -> (x+y=w379:dbl)
          n280 = Bundle By Name(cluster=w377, "Vdc2"=w379) -> (w376:T1)
        }
        frame 774 {
          w391 = 1.0 ("factor 1")
          # "Vdc"
          n281 = call "U8arrayToMeasurement.vi"("factor 2"=w391, "factor 1"=w391, "payload"=w390) -> ("Meas 2"=w388:dbl, "Meas 1"=w389:dbl)
          n282 = Add(x=w389, y=w388) -> (x+y=w384:dbl)
          n283 = Bundle By Name(cluster=w386, "Vdc3"=w384) -> (w385:T1)
        }
        frame 1030 {
          w399 = 1.0 ("factor 1")
          # "Vdc"
          n284 = call "U8arrayToMeasurement.vi"("factor 2"=w399, "factor 1"=w399, "payload"=w398) -> ("Meas 2"=w396:dbl, "Meas 1"=w397:dbl)
          n285 = Add(x=w397, y=w396) -> (x+y=w392:dbl)
          n286 = Bundle By Name(cluster=w393, "Vdc4"=w392) -> (w394:T1)
        }
      }
      n287 = local write "measurements"(w233) -> ()
      n288 = local write "conv"(w235) -> ()
      "CAN IN" <- w237
    }
    n289 = local read "main stop"() -> (w229:bool)
    n290 = node-c288() -> ()  [unwired: 1 in, 1 out]
  }
  n291 = while {
    shift-right: [w404] -> w2
    shift-left: _ -> [w406]
    shift-right: [w405] -> w3
    shift-left: w1 -> [w407]
    tunnel: w4 -> [_]
    stop <- w409 stop-if-true
    w410 = u32 100  # Polling Interval (ms)
    n292 = call "Sync2Tekron.vi"("instrument handle in"=w407, "error in (no error)"=w406) -> ("instrument handle out"=w405:refnum<k15>, "error out"=w404:errorcluster, "Synchronized"=→"Synchronized":bool, "Grandmaster Clock ID"=→"Grandmaster Clock ID":string)  [unwired: 5 in]
    n293 = Wait (ms)(milliseconds to wait=w410) -> ()  [unwired: 1 out]
    n294 = local read "main stop"() -> (w408:bool)
    n295 = Or(x=w404, y=w408) -> (x .or. y?=w409:bool)
  }
  n296 = timed-loop {
    tunnel: w31 -> [w445]
    tunnel: [w444] -> w34
    timing: w25 -> [_]
    timing-out: [_] -> w24
    stop <- w443 stop-if-true
    # "WRITE CAN TO CONVERTER"
    n297 = node-c288() -> ()  [unwired: 1 in, 1 out]
    n298 = Build Array("Clear 1", "Shutdwn 1", "Emergency 1", "To IN OP 1", "SEND sp 1", "To ACT CH 1") -> (w419:bool[])
    n299 = Build Array("Clear 2", "Shutdwn 2", "Emergency 2", "To IN OP  2", "SEND sp 2", "To ACT CH 2") -> (w418:bool[])
    n300 = Build Array("Clear 3", "Shutdwn 3", "Emergency 3", "To IN OP  3", "SEND sp 3", "To ACT CH 3") -> (w417:bool[])
    n301 = Build Array("Clear 4", "Shutdwn 4", "Emergency 4", "To IN OP  4", "SEND sp 4", "To ACT CH 4") -> (w416:bool[])
    n302 = Insert Into Array(array=w419, new element #1=w418, new element #2=w417, new element #3=w416) -> (w415:bool[])  [unwired: 1 in]
    n303 = Search 1D Array(1D array=w415, element=TRUE) -> (index of element=w437:i32)  [unwired: 1 in]
    n304 = Initialize Array(u8 0, 8 ("dimension size")) -> (w451:u8[])
    n305 = To Unsigned Byte Integer(number=w437) -> (unsigned 8bit integer=w441:u8)
    n306 = case shown="4" w441 {
      tunnel: [w465 w468 w475 w482 w489 w496 w503 w510 w517 w523 w530 w537 w544 w551 w558 w565 w572 w582 w600 w618 w636 w651 w658 w665 w672] -> w450
      tunnel: [u32 24 ("identifier") u32 18 ("identifier") u32 40 ("identifier") u32 56 ("identifier") u32 72 ("identifier") u32 24 ("identifier") u32 40 ("identifier") u32 56 ("identifier") u32 72 ("identifier") u32 24 ("identifier") u32 40 ("identifier") u32 56 ("identifier") u32 72 ("identifier") u32 24 ("identifier") u32 40 ("identifier") u32 56 ("identifier") u32 72 ("identifier") w580 w598 w616 w634 u32 24 ("identifier") u32 40 ("identifier") u32 56 ("identifier") u32 72 ("identifier")] -> w449
      tunnel: w451 -> [w463 w468 w473 w480 w487 w495 w502 w509 w516 w524 w531 w538 w545 w552 w559 w566 w573 w579 w597 w615 w633 w652 w659 w666 w673]
      tunnel: [TRUE FALSE TRUE TRUE TRUE TRUE TRUE TRUE TRUE TRUE TRUE TRUE TRUE TRUE TRUE TRUE TRUE w577 w593 w612 w629 TRUE TRUE TRUE TRUE] -> w447
      frame 0 {
        n307 = local write "Clear 1"(FALSE ("Clear")) -> ()
        n308 = Replace Array Subset(array=w463, new element=u8 40 ("new element/subarray"), index=1) -> (w465:u8[])
      }
      frame 99, Default {
      }
      frame 6 {
        n309 = local write "Clear 2"(FALSE ("Clear")) -> ()
        n310 = Replace Array Subset(array=w473, new element=u8 40 ("new element/subarray"), index=1) -> (w475:u8[])
      }
      frame 12 {
        n311 = local write "Clear 3"(FALSE ("Clear")) -> ()
        n312 = Replace Array Subset(array=w480, new element=u8 40 ("new element/subarray"), index=1) -> (w482:u8[])
      }
      frame 18 {
        n313 = local write "Clear 4"(FALSE ("Clear")) -> ()
        n314 = Replace Array Subset(array=w487, new element=u8 40 ("new element/subarray"), index=1) -> (w489:u8[])
      }
      frame 1 {
        n315 = local write "Shutdwn 1"(FALSE ("Shutdwn")) -> ()
        n316 = Replace Array Subset(array=w495, new element=u8 20 ("new element/subarray"), index=0) -> (w496:u8[])
      }
      frame 7 {
        n317 = local write "Shutdwn 2"(FALSE ("Shutdwn")) -> ()
        n318 = Replace Array Subset(array=w502, new element=u8 20 ("new element/subarray"), index=0) -> (w503:u8[])
      }
      frame 13 {
        n319 = local write "Shutdwn 3"(FALSE ("Shutdwn")) -> ()
        n320 = Replace Array Subset(array=w509, new element=u8 20 ("new element/subarray"), index=0) -> (w510:u8[])
      }
      frame 19 {
        n321 = local write "Shutdwn 4"(FALSE ("Shutdwn")) -> ()
        n322 = Replace Array Subset(array=w516, new element=u8 20 ("new element/subarray"), index=0) -> (w517:u8[])
      }
      frame 2 {
        n323 = local write "Emergency 1"(FALSE ("Idc cmd")) -> ()
        n324 = Replace Array Subset(array=w524, new element=u8 30 ("new element/subarray"), index=0) -> (w523:u8[])
      }
      frame 8 {
        n325 = local write "Emergency 2"(FALSE ("Idc cmd")) -> ()
        n326 = Replace Array Subset(array=w531, new element=u8 30 ("new element/subarray"), index=0) -> (w530:u8[])
      }
      frame 14 {
        n327 = local write "Emergency 3"(FALSE ("Idc cmd")) -> ()
        n328 = Replace Array Subset(array=w538, new element=u8 30 ("new element/subarray"), index=0) -> (w537:u8[])
      }
      frame 20 {
        n329 = local write "Emergency 4"(FALSE ("Idc cmd")) -> ()
        n330 = Replace Array Subset(array=w545, new element=u8 30 ("new element/subarray"), index=0) -> (w544:u8[])
      }
      frame 3 {
        n331 = local write "To IN OP 1"(FALSE ("Idc cmd")) -> ()
        n332 = Replace Array Subset(array=w552, new element=u8 2 ("new element/subarray"), index=0) -> (w551:u8[])
      }
      frame 9 {
        n333 = local write "To IN OP  2"(FALSE ("Idc cmd")) -> ()
        n334 = Replace Array Subset(array=w559, new element=u8 2 ("new element/subarray"), index=0) -> (w558:u8[])
      }
      frame 15 {
        n335 = local write "To IN OP  3"(FALSE ("Idc cmd")) -> ()
        n336 = Replace Array Subset(array=w566, new element=u8 2 ("new element/subarray"), index=0) -> (w565:u8[])
      }
      frame 21 {
        n337 = local write "To IN OP  4"(FALSE ("Idc cmd")) -> ()
        n338 = Replace Array Subset(array=w573, new element=u8 2 ("new element/subarray"), index=0) -> (w572:u8[])
      }
      frame 4 {
        (unwired) TRUE
        n339 = case shown="0, Default" u8 0 ("Con_State") {
          tunnel: [w583 w589] -> w582
          tunnel: [u32 16 ("identifier") u32 19 ("identifier")] -> w580
          tunnel: w579 -> [w583 _]
          frame 6 {
            # "PQ mode"
          }
          frame 0, Default {
            # "Vdc Q mode"
            n340 = call "Vdc_lim.vi"("IN Vdc"="Vdc1") -> ("OUT Vdc"=w587:dbl)  [unwired: 10 in]
            n341 = call "Q_limiter.vi"("IN Q"="Qac1") -> ("OUT Q"=w586:dbl)  [unwired: 10 in]
            n342 = call "DoubleToSetpoint.vi"("Double"=w587) -> ("SP"=w591:u8[])
            n343 = call "DoubleToSetpoint.vi"("Double"=w586) -> ("SP"=w590:u8[])
            n344 = Build Array (concatenate)(w591, w590) -> (w589:u8[])
          }
        }
        n345 = local write "SEND sp 1"(FALSE ("SEND sp")) -> ()
        n346 = local read "ON 1"() -> (w576:bool)
        n347 = local read "Ready 1"() -> (w575:bool)
        n348 = Or(x=w576, y=w575) -> (x .or. y?=w577:bool)
      }
      frame 10 {
        (unwired) TRUE
        n349 = case shown="0, Default" u8 0 ("Con_State") {
          tunnel: [w601 w607] -> w600
          tunnel: [u32 32 ("identifier") u32 35 ("identifier")] -> w598
          tunnel: w597 -> [w601 _]
          frame 6 {
            # "PQ mode"
          }
          frame 0, Default {
            # "Vdc Q mode"
            n350 = call "Vdc_lim.vi"("IN Vdc"="Vdc2") -> ("OUT Vdc"=w605:dbl)  [unwired: 10 in]
            n351 = call "Q_limiter.vi"("IN Q"="Qac2") -> ("OUT Q"=w603:dbl)  [unwired: 10 in]
            n352 = call "DoubleToSetpoint.vi"("Double"=w605) -> ("SP"=w609:u8[])
            n353 = call "DoubleToSetpoint.vi"("Double"=w603) -> ("SP"=w608:u8[])
            n354 = Build Array (concatenate)(w609, w608) -> (w607:u8[])
          }
        }
        n355 = local write "SEND sp 2"(FALSE ("SEND sp")) -> ()
        n356 = local read "ON 2"() -> (w594:bool)
        n357 = local read "Ready 2"() -> (w595:bool)
        n358 = Or(x=w594, y=w595) -> (x .or. y?=w593:bool)
      }
      frame 16 {
        (unwired) TRUE
        n359 = case shown="0, Default" u8 0 ("Con_State") {
          tunnel: [w619 w625] -> w618
          tunnel: [u32 48 ("identifier") u32 51 ("identifier")] -> w616
          tunnel: w615 -> [w619 _]
          frame 6 {
            # "PQ mode"
          }
          frame 0, Default {
            # "Vdc Q mode"
            n360 = call "Vdc_lim.vi"("IN Vdc"="Vdc3") -> ("OUT Vdc"=w624:dbl)  [unwired: 10 in]
            n361 = call "Q_limiter.vi"("IN Q"="Qac3") -> ("OUT Q"=w622:dbl)  [unwired: 10 in]
            n362 = call "DoubleToSetpoint.vi"("Double"=w624) -> ("SP"=w627:u8[])
            n363 = call "DoubleToSetpoint.vi"("Double"=w622) -> ("SP"=w626:u8[])
            n364 = Build Array (concatenate)(w627, w626) -> (w625:u8[])
          }
        }
        n365 = local write "SEND sp 3"(FALSE ("SEND sp")) -> ()
        n366 = local read "ON 3"() -> (w613:bool)
        n367 = local read "Ready 3"() -> (w611:bool)
        n368 = Or(x=w613, y=w611) -> (x .or. y?=w612:bool)
      }
      frame 22 {
        (unwired) TRUE
        n369 = case shown="0, Default" u8 0 ("Con_State") {
          tunnel: [w637 w643] -> w636
          tunnel: [u32 64 ("identifier") u32 67 ("identifier")] -> w634
          tunnel: w633 -> [w637 _]
          frame 6 {
            # "PQ mode"
          }
          frame 0, Default {
            # "Vdc Q mode"
            n370 = call "Q_limiter.vi"("IN Q"="Qac4") -> ("OUT Q"=w640:dbl)  [unwired: 10 in]
            n371 = call "Vdc_lim.vi"("IN Vdc"="Vdc4") -> ("OUT Vdc"=w641:dbl)  [unwired: 10 in]
            n372 = call "DoubleToSetpoint.vi"("Double"=w641) -> ("SP"=w645:u8[])
            n373 = call "DoubleToSetpoint.vi"("Double"=w640) -> ("SP"=w644:u8[])
            n374 = Build Array (concatenate)(w645, w644) -> (w643:u8[])
          }
        }
        n375 = local write "SEND sp 4"(FALSE ("SEND sp")) -> ()
        n376 = local read "ON 4"() -> (w630:bool)
        n377 = local read "Ready 4"() -> (w631:bool)
        n378 = Or(x=w630, y=w631) -> (x .or. y?=w629:bool)
      }
      frame 5 {
        n379 = local write "To ACT CH 1"(FALSE ("Idc cmd")) -> ()
        n380 = Replace Array Subset(array=w652, new element=u8 1 ("new element/subarray"), index=0) -> (w651:u8[])
      }
      frame 11 {
        n381 = local write "To ACT CH 2"(FALSE ("Idc cmd")) -> ()
        n382 = Replace Array Subset(array=w659, new element=u8 1 ("new element/subarray"), index=0) -> (w658:u8[])
      }
      frame 17 {
        n383 = local write "To ACT CH 3"(FALSE ("Idc cmd")) -> ()
        n384 = Replace Array Subset(array=w666, new element=u8 1 ("new element/subarray"), index=0) -> (w665:u8[])
      }
      frame 23 {
        n385 = local write "To ACT CH 4"(FALSE ("Idc cmd")) -> ()
        n386 = Replace Array Subset(array=w673, new element=u8 1 ("new element/subarray"), index=0) -> (w672:u8[])
      }
    }
    n387 = Bundle By Name(cluster=T3 {"timestamp"=timestamp(0 s since 1904-01-01), "payload"=[], "identifier"=0, "type"=0, "extended?"=FALSE, "echo?"=FALSE} ("CAN frame 3"), "payload"=w450, "identifier"=w449) -> (w446:T3)
    n388 = local read "main stop"() -> (w443:bool)
    n389 = case shown="True" w447 {
      tunnel: w446 -> [w459 _]
      tunnel: w445 -> [w457 _]
      tunnel: [w456 _] -> w444
      frame True {
        n390 = Build Array(w459) -> (w458:T3[])
        n391 = call-poly <vilib>:"XNET Write.vi"("session in"=w457, "data"=w458) -> ("session out"=w456:refnum<k21>)  [unwired: 12 in, 1 out]
        "CAN OUT" <- w459
      }
      frame False {
      }
    }
    n392 = node-c288() -> ()  [unwired: 1 in, 1 out]
  }
  n393 = call <instrlib>:"niSync Close.vi"("error in (no error)"=w2, "instrument handle"=w3) -> ()  [unwired: 9 in, 1 out]
  n394 = node-c288(w29) -> ()  [unwired: 1 out]
  n395 = node-c288(w24) -> ()  [unwired: 1 out]
  n396 = local write "CAN with Conv"(w32) -> ()
  n397 = call <vilib>:"XNET Stop.vi"("session in"=w35) -> ()  [unwired: 13 in, 2 out]
  n398 = call <vilib>:"XNET Stop.vi"("session in"=w34) -> ()  [unwired: 13 in, 2 out]
  n399 = node-c288(w22) -> ()  [unwired: 1 out]
  n400 = UDP Close(connection ID=w17, 8:w16) -> ()  [unwired: 2 out]
  "Measurements" <- w7
  "CAN with Conv" <- w7
  "logging" <- w7
  "Ready 1" <- w7
  "OFF 1" <- w7
  "Ready 2" <- w7
  "ON 2" <- w7
  "OFF 2" <- w7
  "Ready 4" <- w7
  "ON 4" <- w7
  "OFF 4" <- w7
  "ON 3" <- w7
  "Ready 3" <- w7
  "OFF 3" <- w7
  "Fault 1" <- w7
  "Error 1" <- w7
  "Fault 2" <- w7
  "Error 2" <- w7
  "Fault 3" <- w7
  "Error 3" <- w7
  "Fault 4" <- w7
  "Error 4" <- w7
